vi "read bmp string.vi"(8 "error in":errorcluster, 11 "file string":string) -> (0 "error out":errorcluster, 2 "found":bool, 3 "<bmp> string":string)   [LabVIEW 2018, in "Data Parser.lvclass"]
uses:
  Data Parser.lvclass
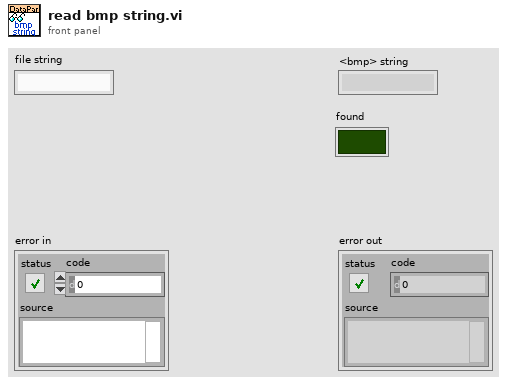
[diagram p1: front panel]
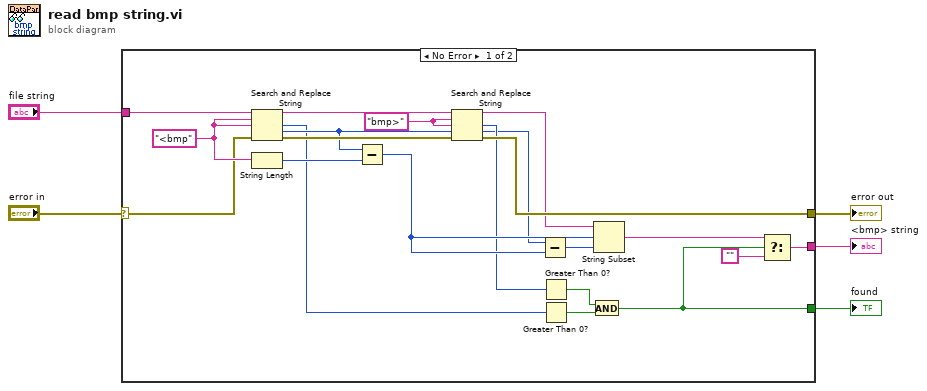
[diagram p0: block diagram]
diagram:
  n1 = case shown="No Error" "error in" {
    selector: "error in" -> [w6 w27]
    tunnel: "file string" -> [w26 _]
    tunnel: [w25 w27] -> w4
    tunnel: [w14 _] -> w3
    tunnel: [w9 _] -> w1
    frame No Error {
      w19 = "bmp>" ("format string")
      w7 = "<bmp" ("format string")
      n2 = Search and Replace String(input string=w26, search string=w7, replace string=w7, error in=w6) -> (result string=w24:string, number of replacements=w16:i32, offset past replacement=w21:i32, error out=w23:errorcluster)  [unwired: 4 in]
      n3 = String Length(string=w7) -> (length=w20:i32)
      n4 = Subtract(x=w21, y=w20) -> (x-y=w18:i32)
      n5 = Search and Replace String(input string=w24, search string=w19, replace string=w19, offset=w21, error in=w23) -> (result string=w22:string, number of replacements=w12:i32, offset past replacement=w8:i32, error out=w25:errorcluster)  [unwired: 3 in]
      n6 = Subtract(x=w8, y=w18) -> (x-y=w17:i32)
      n7 = Greater Than 0?(x=w12) -> (x > 0?=w11:bool)
      n8 = Greater Than 0?(x=w16) -> (x > 0?=w10:bool)
      n9 = And(x=w11, y=w10) -> (x .and. y?=w9:bool)
      n10 = String Subset(string=w22, offset (0)=w18, length (rest)=w17) -> (substring=w13:string)
      n11 = Select(t=w13, s=w9, f="") -> (s? t:f=w14:string)
    }
    frame Error {
    }
  }
  "error out" <- w4
  "<bmp> string" <- w3
  "found" <- w1
